vi "String - String to Ctl.vi"(10 "String":string, 11 "Reference In":refnum<vi>) -> (3 "Reference Out":refnum<vi>)   [LabVIEW 2013]
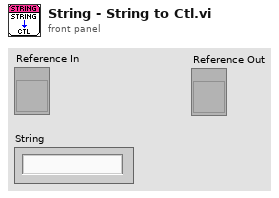
[diagram p1: front panel]
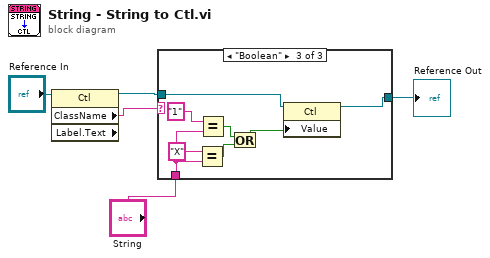
[diagram p0: block diagram]
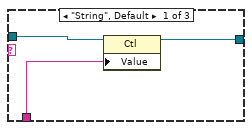
[diagram p2: hidden frame]
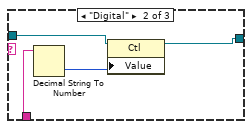
[diagram p3: hidden frame]
diagram:
  n1 = property class="Ctl" props=["ClassName", "Label", "Text"](reference="Reference In") -> (reference out=w4:refnum<vi>, "ClassName"=w5:string)  [unwired: 1 in, 2 out]
  n2 = case shown="\"Boolean\"" w5 {
    tunnel: "String" -> [w8 w12 w18]
    tunnel: w4 -> [w7 w10 w15]
    tunnel: [w6 w9 w13] -> w1
    frame "String", Default {
      n3 = property class="Ctl"(reference=w7, "Value"=w8) -> (reference out=w6:refnum<vi>)  [unwired: 1 in, 1 out]
    }
    frame "Digital" {
      n4 = Decimal String To Number(string=w12) -> (number=w11:i32)  [unwired: 2 in, 1 out]
      n5 = property class="Ctl"(reference=w10, "Value"=w11) -> (reference out=w9:refnum<vi>)  [unwired: 1 in, 1 out]
    }
    frame "Boolean" {
      n6 = Equal?(x="X", y=w18) -> (x = y?=w16:bool)
      n7 = Equal?(x="1", y=w18) -> (x = y?=w19:bool)
      n8 = Or(x=w19, y=w16) -> (x .or. y?=w14:bool)
      n9 = property class="Ctl"(reference=w15, "Value"=w14) -> (reference out=w13:refnum<vi>)  [unwired: 1 in, 1 out]
    }
  }
  "Reference Out" <- w1
